vi "GlobalCameraDebugTemperature.vi"() -> ()   [LabVIEW 2011]
panel:
  in  "temperature":i32=-70
  in  "Debug":enum16{"Debug", "Normal"}(ring)=enum."Normal"
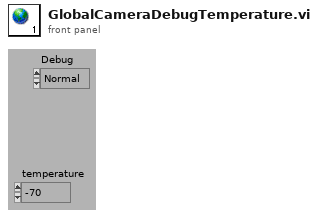
[diagram p1: front panel]
diagram:
